vi "Read the Internal Project Home.vi"(4 "Error In":errorcluster) -> (0 "Error Out":errorcluster, 3 "Internal Home Path":path)   [LabVIEW 2014, in "Path Utilities.lvlib"]
uses:
  Path Utilities.lvlib
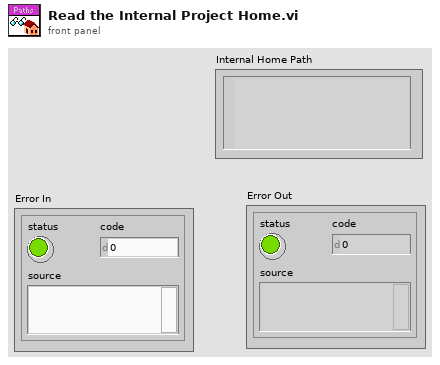
[diagram p1: front panel]
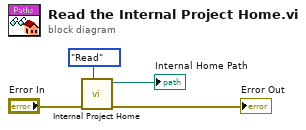
[diagram p0: block diagram]
diagram:
  n1 = call "Internal Project Home.vi"("Function"=enum16{"Read", "Write"}."Read", "Error In"="Error In") -> ("Error Out"=→"Error Out":errorcluster, "Internal Home Path"=→"Internal Home Path":path)  [unwired: 5 in]
